vi "SC10 example.vi"() -> ()   [LabVIEW 2013]
uses:
  <instrlib>/Thorlabs_SC10/Public/Configure/Mode.ctl
  <instrlib>/Thorlabs_SC10/Public/Configure/Trigger Mode.ctl
  <instrlib>/Thorlabs_SC10/Thorlabs_SC10.lvlib
panel:
  out "ID":string
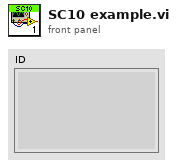
[diagram p1: front panel]
types:
  T1 = typedef "Thorlabs_SC10.lvlib/Trigger Mode.ctl" = enum16{"Internal", "External"}
  T2 = typedef "Thorlabs_SC10.lvlib/Mode.ctl" = enum16{"manual", "auto", "single", "repeat", "external gate"}
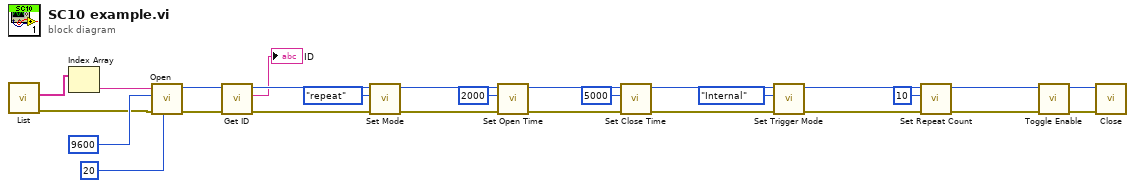
[diagram p0: block diagram]
diagram:
  n1 = call <instrlib>:"List.vi"() -> ("error out"=w3:errorcluster, "COM ports"=w2:string[])  [unwired: 10 in]
  n2 = Index Array(array=w2) -> (element=w1:string)  [unwired: 1 in]
  n3 = call <instrlib>:"Open.vi"("timeout"=20, "error in (no error)"=w3, "nbaud"=9600, "Serial Port"=w1) -> ("error out"=w6:errorcluster, "hDevice"=w27:i32)  [unwired: 5 in, 1 out]
  n4 = call <instrlib>:"Get ID.vi"("error in (no error)"=w6, "hdl"=w27) -> ("error out"=w5:errorcluster, "ID"=→"ID":string, "hdl out"=w7:i32)  [unwired: 7 in]
  n5 = call <instrlib>:"Set Mode.vi"("error in (no error)"=w5, "Mode"=Mode."repeat" ("Cycle Mode?"), "hdl"=w7) -> ("error out"=w19:errorcluster, "hdl out"=w25:i32)  [unwired: 7 in]
  n6 = call <instrlib>:"Set Open Time.vi"("error in (no error)"=w19, "Open time (ms)"=2000, "hdl"=w25) -> ("error out"=w17:errorcluster, "hdl out"=w21:i32)  [unwired: 7 in]
  n7 = call <instrlib>:"Set Close Time.vi"("error in (no error)"=w17, "Close time (ms)"=5000, "hdl"=w21) -> ("error out"=w15:errorcluster, "hdl out"=w22:i32)  [unwired: 7 in]
  n8 = call <instrlib>:"Set Trigger Mode.vi"("error in (no error)"=w15, "Trigger Mode"=Trigger_Mode."Internal", "hdl"=w22) -> ("error out"=w11:errorcluster, "hdl out"=w13:i32)  [unwired: 7 in]
  n9 = call <instrlib>:"Set Repeat Count.vi"("error in (no error)"=w11, "Repeat Count"=10, "hdl"=w13) -> ("error out"=w9:errorcluster, "hdl out"=w14:i32)  [unwired: 7 in]
  n10 = call <instrlib>:"Toggle Enable.vi"("error in (no error)"=w9, "hdl"=w14) -> ("error out"=w8:errorcluster, "hdl out"=w10:i32)  [unwired: 8 in]
  n11 = call <instrlib>:"Close.vi"("error in (no error)"=w8, "hDevice"=w10) -> ()  [unwired: 9 in, 1 out]
